vi "send_internal_trigger.vi"(7 "unique insertion?":bool, 8 "error in (no error)":errorcluster, 10 "trigger":T1, 11 "DL090216Display in":refnum<class "DisplayDL090216.lvclass">) -> (0 "error out":errorcluster, 3 "DL090216Display out":refnum<class "DisplayDL090216.lvclass">)   [LabVIEW 2010, in "DisplayDL090216.lvclass"]
uses:
  DisplayDL090216.lvclass
  action_enum.ctl
  common/classes/GenericToplevelComponent/GenericToplevelComponent/trigger_type_enum.ctl
  common/classes/ErrorController/ErrorController/class_data.vi
  common/classes/ErrorController/ErrorController/ErrorController.lvclass
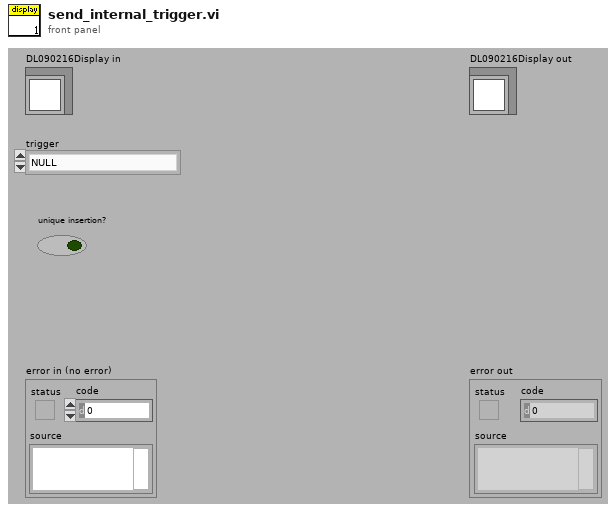
[diagram p1: front panel]
types:
  T1 = typedef "DisplayDL090216.lvclass/action_enum.ctl" = enum16{"NULL", "initialise", "terminate", "fetch", "process", "display", "register as observer"}
  T2 = typedef "trigger_type_enum.ctl" = enum8{"external", "internal", "common"}
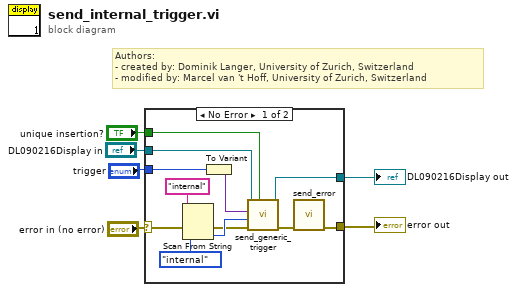
[diagram p0: block diagram]
diagram:
  # "Authors: \n- created by: Dominik Langer, University of Zurich, Switzerland\n- modified by: Marcel van 't Hoff, University of Zurich, Switzerland"
  n1 = case shown="No Error" "error in (no error)" {
    selector: "error in (no error)" -> [w9 w20]
    tunnel: [w17 w20] -> w3
    tunnel: [w12 w19] -> w4
    tunnel: "DL090216Display in" -> [w15 w19]
    tunnel: "trigger" -> [w18 _]
    tunnel: "unique insertion?" -> [w13 _]
    frame No Error {
      n2 = Scan From String(input string="internal", error in=w9, default 1=trigger_type_enum."internal" ("trigger type")) -> (error out=w8:errorcluster, output 1=w10:T2)  [unwired: 2 in, 2 out]
      n3 = To Variant(anything=w18) -> (Variant=w16:variant)
      n4 = call-dynamic "send_generic_trigger.vi"("ensure unique insertion?"=w13, "error in (no error)"=w8, "trigger type"=w10, "trigger variant"=w16, "GenericToplevelComponent in"=w15) -> ("error out"=w14:errorcluster, "GenericToplevelComponent out"=w12:refnum<class "DisplayDL090216.lvclass">)  [unwired: 3 in, 2 out]
      n5 = call "send_error.vi"("error in (no error)"=w14) -> ("error out"=w17:errorcluster)  [unwired: 10 in]
    }
    frame Error {
    }
  }
  "error out" <- w3
  "DL090216Display out" <- w4
